vi "Execute.vi"(8 "Error In":errorcluster, 11 "Audio Analyzer In":refnum<class "Audio Analyzer.lvclass">) -> (0 "Error Out":errorcluster, 3 "Audio Analyzer Out":refnum<class "Audio Analyzer.lvclass">)   [LabVIEW 2019, in "Audio Analyzer.lvclass"]
uses:
  Audio Analyzer.lvclass
  C:/Users/goo13/Documents/GIT Local/myDashBoard/Source/RT/Process/Process.lvclass
  Private/Controls/State.ctl
  Process/Process.lvclass
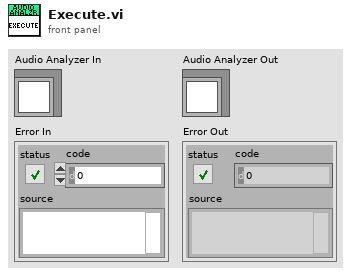
[diagram p1: front panel]
types:
  T1 = typedef "Audio Analyzer.lvclass/State.ctl" = enum16{"Initialize", "Wait for command", "Start Audio Analyzer", "Analyze Audio", "Stop Audio Analyzer", "Shutdown"}
  T2 = typedef "Process.lvclass/Process Message.ctl" = cluster{"Command":string, "Data":variant}
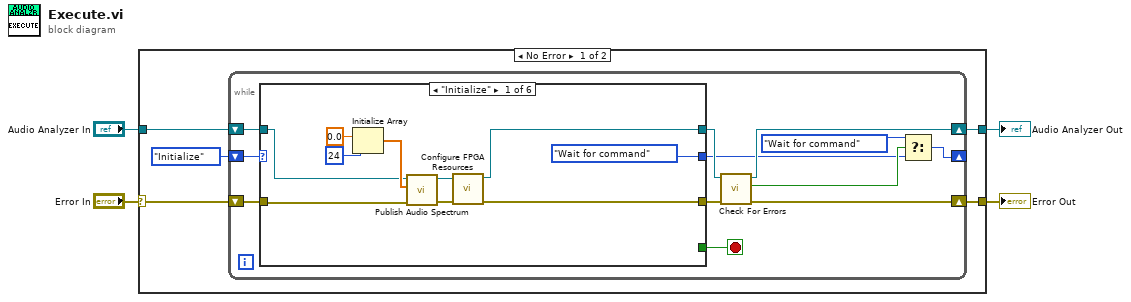
[diagram p0: block diagram]
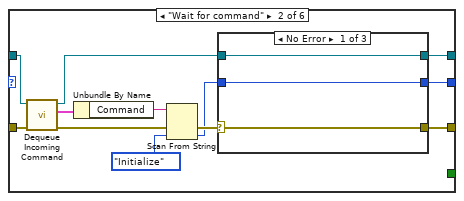
[diagram p2: hidden frame]
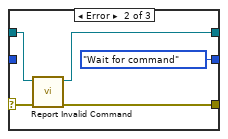
[diagram p3: hidden frame]
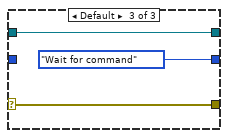
[diagram p4: hidden frame]
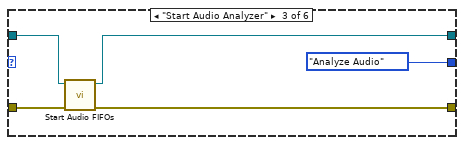
[diagram p5: hidden frame]
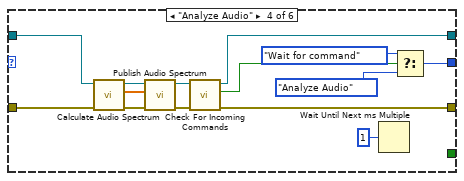
[diagram p6: hidden frame]
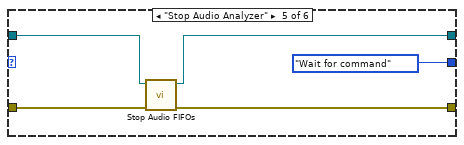
[diagram p7: hidden frame]
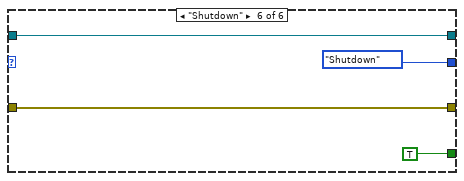
[diagram p8: hidden frame]
diagram:
  n1 = case shown="No Error" "Error In" {
    selector: "Error In" -> [w8 w84]
    tunnel: [w9 w84] -> w3
    tunnel: "Audio Analyzer In" -> [w7 w83]
    tunnel: [w6 w83] -> w1
    frame No Error {
      n2 = while {
        shift-right: [w10] -> w9
        shift-left: w8 -> [w21]
        shift-right: [w15] -> w6
        shift-left: w7 -> [w20]
        shift-right: [w11] -> _
        shift-left: State."Initialize" ("State") -> [w19]
        stop <- w18 stop-if-true
        n3 = case shown="\"Initialize\"" w19 {
          tunnel: w21 -> [w22 w43 w57 w73 w76 w81]
          tunnel: w20 -> [w25 w42 w58 w72 w77 w82]
          tunnel: [w31 w33 w55 w71 w75 w82] -> w16
          tunnel: [w30 w32 w56 w66 w74 w81] -> w17
          tunnel: [State."Wait for command" ("State") w35 State."Analyze Audio" ("State") w69 State."Wait for command" ("State") State."Shutdown" ("State")] -> w13
          tunnel: [_ _ _ _ _ TRUE] -> w18
          frame "Initialize" {
            n4 = Initialize Array(0.0 ("element"), 24 ("dimension size")) -> (w26:dbl[])
            n5 = call "Publish Audio Spectrum.vi"("Error In"=w22, "Audio Spectrum"=w26, "Audio Analyzer In"=w25) -> ("Error Out"=w23:errorcluster, "Audio Analyzer Out"=w24:refnum<class "Audio Analyzer.lvclass">)  [unwired: 7 in]
            n6 = call "Configure FPGA Resources.vi"("Error In"=w23, "Audio Analyzer In"=w24) -> ("Error Out"=w30:errorcluster, "Audio Analyzer Out"=w31:refnum<class "Audio Analyzer.lvclass">)  [unwired: 8 in]
          }
          frame "Wait for command" {
            n7 = call "Dequeue Incoming Command.vi"("Error In"=w43, "Process In"=w42) -> ("Error Out"=w38:errorcluster, "Process Message"=w41:T2, "Process Out"=w34:refnum<class "Audio Analyzer.lvclass">)  [unwired: 6 in, 1 out]
            n8 = Unbundle By Name(w41) -> ("Command"=w40:string)
            n9 = Scan From String(input string=w40, error in=w38, default 1=State."Initialize" ("State")) -> (error out=w37:errorcluster, output 1=w36:T1)  [unwired: 2 in, 2 out]
            n10 = case shown="No Error" w37 {
              selector: w37 -> [w44 w48 w53]
              tunnel: w36 -> [w46 _ _]
              tunnel: [w46 State."Wait for command" ("State") State."Wait for command" ("State")] -> w35
              tunnel: w34 -> [w45 w50 w54]
              tunnel: [w45 w49 w54] -> w33
              tunnel: [w44 w47 w53] -> w32
              frame No Error {
              }
              frame Error {
                n11 = call "Report Invalid Command.vi"("Error In"=w48, "Process In"=w50) -> ("Error Out"=w47:errorcluster, "Process Out"=w49:refnum<class "Audio Analyzer.lvclass">)  [unwired: 8 in]
              }
              frame Default {
              }
            }
          }
          frame "Start Audio Analyzer" {
            n12 = call "Start Audio FIFOs.vi"("Error In"=w57, "Audio Analyzer In"=w58) -> ("Error Out"=w56:errorcluster, "Audio Analyzer Out"=w55:refnum<class "Audio Analyzer.lvclass">)  [unwired: 8 in]
          }
          frame "Analyze Audio" {
            n13 = call "Calculate Audio Spectrum.vi"("Error In"=w73, "Audio Analyzer In"=w72) -> ("Error Out"=w64:errorcluster, "Audio Spectrum"=w61:dbl[], "Audio Analyzer Out"=w65:refnum<class "Audio Analyzer.lvclass">)  [unwired: 6 in, 1 out]
            n14 = call "Publish Audio Spectrum.vi"("Error In"=w64, "Audio Spectrum"=w61, "Audio Analyzer In"=w65) -> ("Error Out"=w62:errorcluster, "Audio Analyzer Out"=w63:refnum<class "Audio Analyzer.lvclass">)  [unwired: 7 in]
            n15 = call "Check For Incoming Commands.vi"("Error In"=w62, "Process In"=w63) -> ("Error Out"=w66:errorcluster, "New Command(s)"=w70:bool, "Process Out"=w71:refnum<class "Audio Analyzer.lvclass">)  [unwired: 7 in]
            n16 = Wait Until Next ms Multiple(millisecond multiple=u32 1) -> ()  [unwired: 1 out]
            n17 = Select(t=State."Wait for command" ("State"), s=w70, f=State."Analyze Audio" ("State")) -> (s? t:f=w69:T1)
          }
          frame "Stop Audio Analyzer" {
            n18 = call "Stop Audio FIFOs.vi"("Error In"=w76, "Audio Analyzer In"=w77) -> ("Error Out"=w74:errorcluster, "Audio Analyzer Out"=w75:refnum<class "Audio Analyzer.lvclass">)  [unwired: 8 in]
          }
          frame "Shutdown" {
          }
        }
        n19 = call "Check For Errors.vi"("Error In"=w17, "Process In"=w16) -> ("Error Out"=w10:errorcluster, "Error Detected"=w14:bool, "Process Out"=w15:refnum<class "Audio Analyzer.lvclass">)  [unwired: 7 in]
        n20 = Select(t=State."Wait for command", s=w14, f=w13) -> (s? t:f=w11:T1)
      }
    }
    frame Error {
    }
  }
  "Error Out" <- w3
  "Audio Analyzer Out" <- w1
